vi "Compiled Get Node Frames.Incoming.vi"(8 "error in (no error)":errorcluster, 9 "Cluster":refnum<k21>, 10 "Section Ref in":T5 format="%.0x", 11 "Device Ref in":T5=18446744073709551615 format="%.0x") -> (0 "error out":errorcluster, 2 "Incoming.Settings":T1 {"Timing.Refs"."Data Reference" format="%.0x"; "Data.Refs"."Data Reference" format="%.0x"}, 3 "Device Ref out":T5=18446744073709551615 format="%.0x")   [LabVIEW 2023, in "J1939 Addon System Explorer.lvlib"]
uses:
  J1939 Addon System Explorer.lvlib
  <vilib>/NI VeriStand/Custom Device API/Custom Device Item Ref.ctl
  Addon Shared/Types/Incoming Settings.ctl
  Addon Shared/Types/Incoming Frame Settings.ctl
  <vilib>/NI VeriStand/Custom Device API/Block Data Reference.ctl
  <vilib>/NI VeriStand/Custom Device API/Data Reference.ctl
  <vilib>/NI VeriStand/Custom Device API/Data Access Type.ctl
  Support Libraries/J1939 Utilities/SubVIs/Convert CAN Arb ID to J1939 ID.vi
  Addon Shared/SubVIs/Constants.vi
  <vilib>/NI VeriStand/Custom Device API/Custom Device API.lvlib
  Addon Shared/J1939 Addon Shared.lvlib
  Support Libraries/J1939 Utilities/J1939 Utilities.lvlib
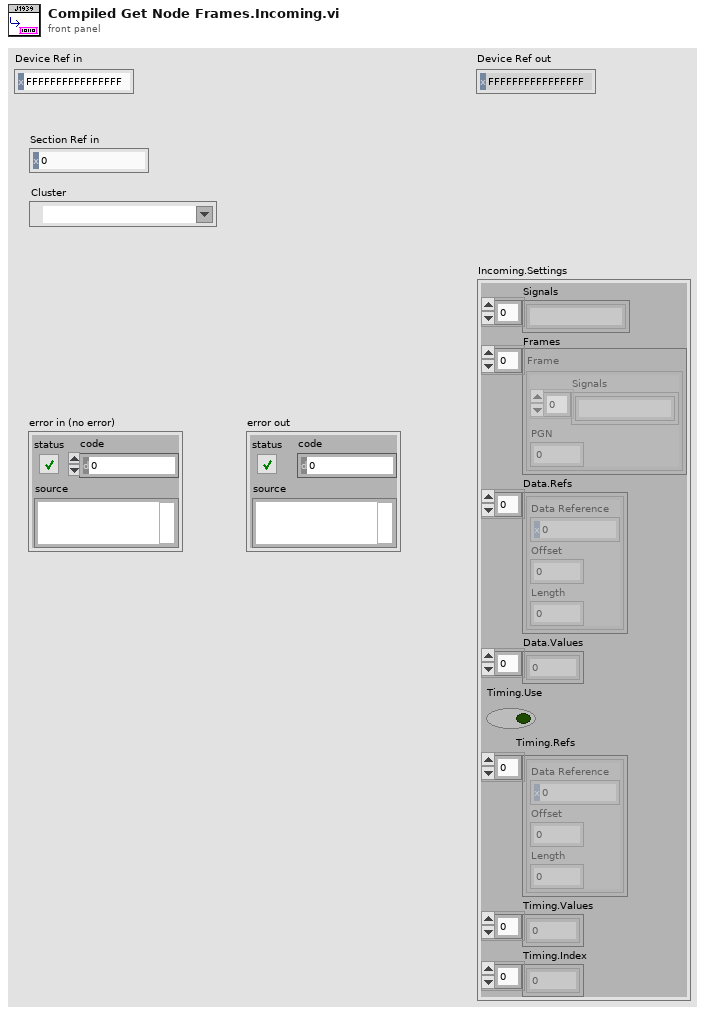
[diagram p1: front panel]
types:
  T1 = typedef "J1939 Addon Shared.lvlib/Incoming Settings.ctl" = cluster{"Signals":string[], "Frames":T2[], "Data.Refs":T3[], "Data.Values":dbl[], "Timing.Use":bool, "Timing.Refs":T3[], "Timing.Values":dbl[], "Timing.Index":i32[]}
  T2 = typedef "J1939 Addon Shared.lvlib/Incoming Frame Settings.ctl" = cluster{"Signals":string[], "PGN":u32}
  T3 = typedef "Custom Device API.lvlib/Block Data Reference.ctl" = cluster{"Data Reference":T4, "Offset":u64, "Length":u64}
  T4 = typedef "Custom Device API.lvlib/Data Reference.ctl" = i32
  T5 = typedef "Custom Device API.lvlib/Custom Device Item Ref.ctl" = u64
  T6 = typedef "Custom Device API.lvlib/Data Access Type.ctl" = enum16{"Read", "Write"}
  T7 = typedef "Custom Device API.lvlib/Custom Device Item Info.ctl" = cluster{"Name":string, "Is Channel":bool, "GUID":string, "Is Waveform":bool}
  T8 = typedef "J1939 Addon Shared.lvlib/Frame.Settings.ctl" = cluster{"ID":u32, "Disable Transmission":bool, "Disable Transmission Ref":T5, "Transmit Trigger":T9, "Transmit Trigger Ref":T5}
  T9 = typedef "J1939 Addon Shared.lvlib/Outgoing Event Trigger Types.ctl" = enum16{"Channel value change", "Trigger channel (not zero)", "Channel value change or trigger channel (not zero)", "Trigger channel (any value change)", "Channel value change or trigger channel (any value change)"}
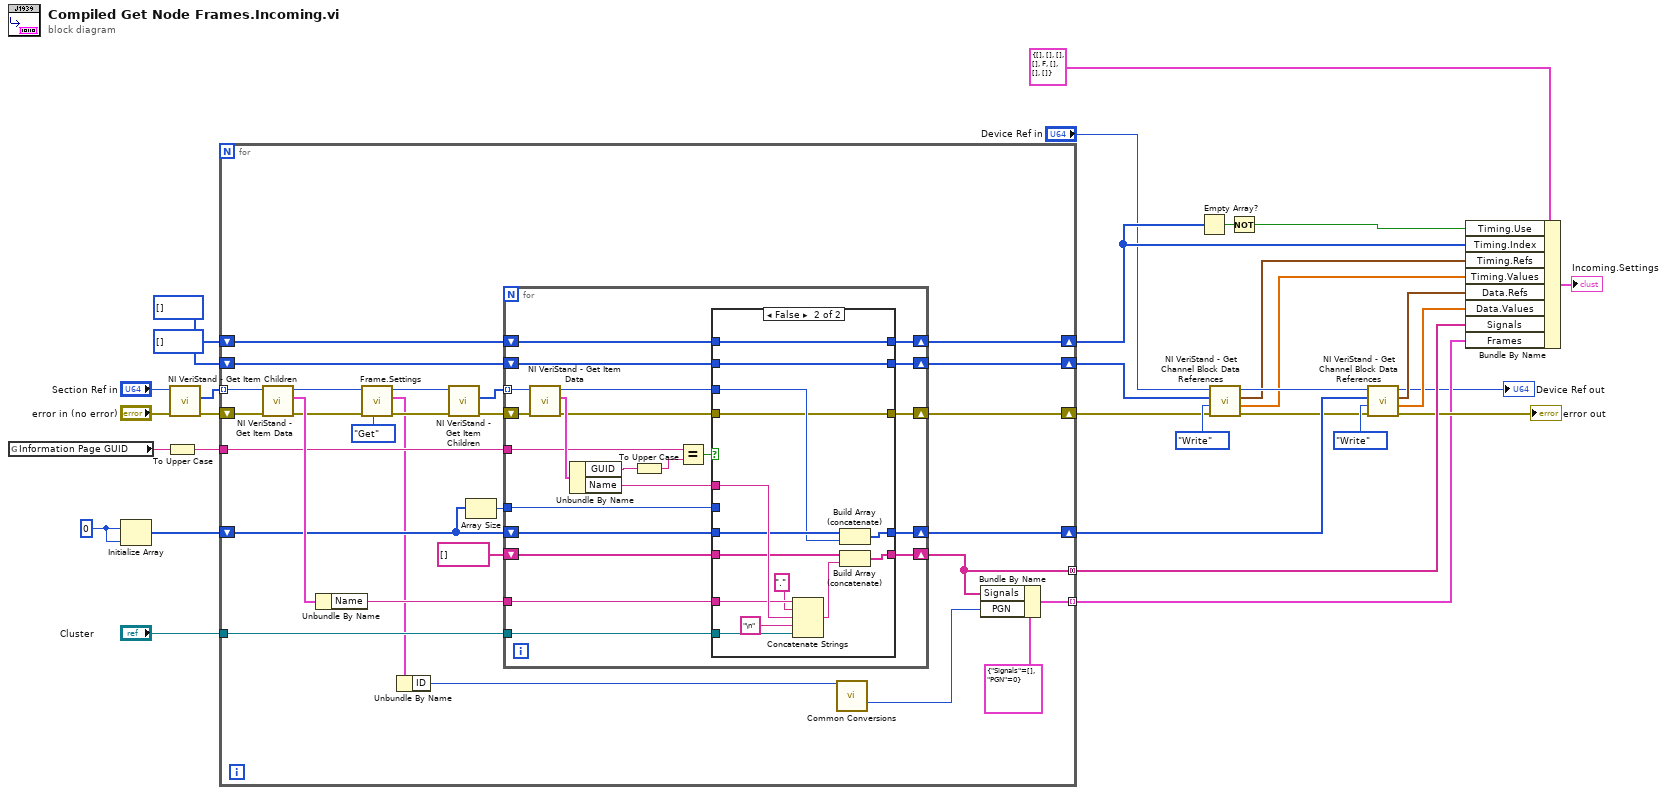
[diagram p0: block diagram]
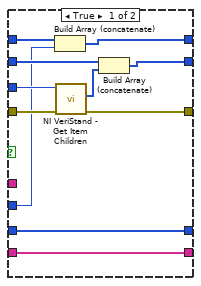
[diagram p2: hidden frame]
diagram:
  w32 = T4 0 ("Channel Data Reference")
  n1 = global read "Constants.vi" "Information Page GUID"() -> (w25:string)
  n2 = Initialize Array(w32, w32) -> (w31:T4[])
  n3 = To Upper Case(1:w25) -> (0:w24:string)
  n4 = call <vilib>:"NI VeriStand - Get Item Children.vi"("error in (no error)"="error in (no error)", "Item Ref in"="Section Ref in") -> ("error out"=w28:errorcluster, "Child Refs"=w30:T5[])  [unwired: 6 in, 2 out]
  n5 = for {
    shift-right: [w49] -> w12
    shift-left: w28 -> [w54]
    tunnel: w30 -> [w55] mode=indexing
    shift-right: [w57] -> w18
    shift-left: w31 -> [w38]
    tunnel: [w41] -> w20 mode=concatenating
    tunnel: "Cluster" -> [w48]
    tunnel: [w46] -> w14 mode=indexing
    tunnel: w24 -> [w43]
    shift-right: [w40] -> w9
    shift-left: T5[] [] ("Child Refs") -> [w39]
    shift-right: [w35] -> w4
    shift-left: i32[] [] ("Child Refs") -> [w36]
    n6 = call <vilib>:"NI VeriStand - Get Item Data.vi"("error in (no error)"=w54, "Item Ref in"=w55) -> ("error out"=w51:errorcluster, "Item Info"=w53:T7, "Item Ref out"=w52:T5)  [unwired: 6 in, 1 out]
    n7 = Unbundle By Name(w53) -> ("Name"=w50:string)
    n8 = call "Frame.Settings.vi"("Action"=enum8{"Get", "Set"}."Get", "error in (no error)"=w51, "Item Ref in"=w52) -> ("error out"=w60:errorcluster, "Frame.Settings"=w34:T8, "Item Ref out"=w59:T5)  [unwired: 6 in]
    n9 = Unbundle By Name(w34) -> ("ID"=w33:u32)
    n10 = call <vilib>:"NI VeriStand - Get Item Children.vi"("error in (no error)"=w60, "Item Ref in"=w59) -> ("error out"=w58:errorcluster, "Child Refs"=w56:T5[])  [unwired: 6 in, 2 out]
    n11 = Array Size(array=w38) -> (size(s)=w37:i32)
    n12 = for {
      shift-right: [w66] -> w49
      shift-left: w58 -> [w81]
      tunnel: w56 -> [w82] mode=indexing
      shift-right: [w76] -> w57
      shift-left: w38 -> [w77]
      tunnel: w50 -> [w75]
      tunnel: w48 -> [w73]
      tunnel: w43 -> [w72]
      shift-right: [w78] -> w41
      shift-left: string[] [] ("Signals") -> [w68]
      shift-right: [w65] -> w40
      shift-left: w39 -> [w64]
      tunnel: w37 -> [w63]
      shift-right: [w61] -> w35
      shift-left: w36 -> [w62]
      n13 = call <vilib>:"NI VeriStand - Get Item Data.vi"("error in (no error)"=w81, "Item Ref in"=w82) -> ("error out"=w67:errorcluster, "Item Info"=w80:T7, "Item Ref out"=w74:T5)  [unwired: 6 in, 1 out]
      n14 = Unbundle By Name(w80) -> ("GUID"=w71:string, "Name"=w79:string)
      n15 = To Upper Case(1:w71) -> (0:w70:string)
      n16 = Equal?(x=w72, y=w70) -> (x = y?=w69:bool)
      n17 = case shown="False" w69 {
        tunnel: w79 -> [_ w107]
        tunnel: [w93 w97] -> w78
        tunnel: w77 -> [w92 w105]
        tunnel: [w92 w104] -> w76
        tunnel: w75 -> [_ w103]
        tunnel: w74 -> [w90 w101]
        tunnel: w73 -> [_ w100]
        tunnel: w68 -> [w93 w99]
        tunnel: w67 -> [w91 w96]
        tunnel: [w89 w96] -> w66
        tunnel: [w86 w95] -> w65
        tunnel: w64 -> [w88 w95]
        tunnel: w63 -> [w85 _]
        tunnel: w62 -> [w84 w94]
        tunnel: [w83 w94] -> w61
        frame True {
          n18 = Build Array (concatenate)(w84, w85) -> (w83:i32[])
          n19 = call <vilib>:"NI VeriStand - Get Item Children.vi"("error in (no error)"=w91, "Item Ref in"=w90) -> ("error out"=w89:errorcluster, "Child Refs"=w87:T5[])  [unwired: 6 in, 2 out]
          n20 = Build Array (concatenate)(w88, w87) -> (w86:T5[])
        }
        frame False {
          n21 = Concatenate Strings(w103, "." ("string"), w107, "\n" ("string"), w100) -> (w98:string)
          n22 = Build Array (concatenate)(w105, w101) -> (w104:T5[])
          n23 = Build Array (concatenate)(w99, w98) -> (w97:string[])
        }
      }
    }
    n24 = call-poly "Common Conversions.vi"("Arb ID"=w33) -> ("PGN"=w44:u32)  [unwired: 11 in, 3 out]
    n25 = Bundle By Name(cluster=T2 {"Signals"=[], "PGN"=0} ("Frame"), "Signals"=w41, "PGN"=w44) -> (w46:T2)
  }
  n26 = Empty Array?(array=w4) -> (empty?=w6:bool)
  n27 = call <vilib>:"NI VeriStand - Get Channel Block Data References.vi"("error in (no error)"=w12, "Access"=Data_Access_Type."Write", "Channel Refs"=w9, "Device Ref in"="Device Ref in") -> ("error out"=w11:errorcluster, "Values Array"=w8:dbl[], "Block Data Refs"=w7:T3[], "Device Ref out"=w10:T5)  [unwired: 4 in]
  n28 = Not(x=w6) -> (.not. x?=w5:bool)
  n29 = call <vilib>:"NI VeriStand - Get Channel Block Data References.vi"("error in (no error)"=w11, "Access"=Data_Access_Type."Write", "Channel Refs"=w18, "Device Ref in"=w10) -> ("error out"=→"error out":errorcluster, "Values Array"=w16:dbl[], "Block Data Refs"=w15:T3[], "Device Ref out"=→"Device Ref out":T5)  [unwired: 4 in]
  n30 = Bundle By Name(cluster=T1 {"Signals"=[], "Frames"=[], "Data.Refs"=[], "Data.Values"=[], "Timing.Use"=FALSE, "Timing.Refs"=[], "Timing.Values"=[], "Timing.Index"=[]} ("Incoming"), "Timing.Use"=w5, "Timing.Index"=w4, "Timing.Refs"=w7, "Timing.Values"=w8, "Data.Refs"=w15, "Data.Values"=w16, "Signals"=w20, "Frames"=w14) -> (→"Incoming.Settings":T1)
